vi "FlatToRichcalculator_AddRequest.vi"(5 "OutputClusterType":T1, 11 "InputCluster":T2) -> (3 "OutputCluster":T1)   [LabVIEW 2025, in "calculator_client.lvlib"]
uses:
  calculator_AddRequest_Flat.ctl
  calculator_AddRequest.ctl
  calculator_client.lvlib
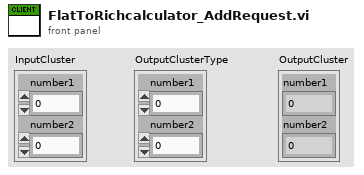
[diagram p1: front panel]
types:
  T1 = typedef "calculator_client.lvlib/calculator_AddRequest.ctl" = cluster{"number1":dbl, "number2":dbl}
  T2 = typedef "calculator_client.lvlib/calculator_AddRequest_Flat.ctl" = cluster{"number1":dbl, "number2":dbl}
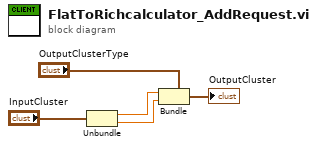
[diagram p0: block diagram]
diagram:
  n1 = Unbundle "Unbundle"("InputCluster") -> ("number1"=w2:dbl, "number2"=w1:dbl)
  n2 = Bundle "Bundle"(cluster="OutputClusterType", "number1"=w2, "number2"=w1) -> (→"OutputCluster":T1)
